vi "SMR_LabVIEW_V7.3.vi"() -> ()   [LabVIEW 2025]
uses:
  <vilib>/DAQmx/write.llb/DAQmx Write (Analog DBL 1Chan 1Samp).vi
  <vilib>/DAQmx/read.llb/DAQmx Read (Analog 1D DBL NChan 1Samp).vi
  <vilib>/DAQmx/create/channels.llb/DAQmx Create Channel (AI-Temperature-Thermocouple).vi
  <vilib>/DAQmx/create/channels.llb/DAQmx Create Channel (AI-Voltage-Basic).vi
  <vilib>/DAQmx/create/channels.llb/DAQmx Create Channel (AO-Voltage-Basic).vi
  <vilib>/DAQmx/miscellaneous.llb/DAQmx Fill In Error Info.vi
  <vilib>/addons/control/pid/pid.llb/PID (DBL).vi
  <vilib>/addons/control/pid/NI_PID_pid.lvlib
panel:
  out "Current Run Folder":path
  in  "Log Root Folder":path=path "C:/Users/LocalUser/Documents/GitHub/thermal-loop/resources/v0.1.1/data/001"
  out "Raw NI9201 \nVoltage Display":T1
  in  "Loop Period (ms)":dbl=1000.0
  in  "Stop":bool
  out "Auto Steady State Threshold (deg C/min)":dbl
  out "Max dT/dt (deg C/min)":dbl
  out "Temp Change Rate (deg C/min)":dbl
  out "5-Min Baseline Complete":bool
  out "Rate Window Ready":bool
  out "Steady State":bool
  in  "Voltage Limit (V)":dbl=10.0
  in  "Temperature Limit (C)":dbl=50.0
  in  "Pressure Limit (psi)":dbl=15.0
  out "Max Voltage":bool
  out "Max Temperature":bool
  out "Max Pressure":bool
  out "Heat Exchanger Pressure History":dbl(graph)
  out "Main Loop Pressure History":T2(graph)
  out "Overall Avg Pressure (psi)":dbl
  out "Heat Exchanger Pressure P6 (psi)":dbl
  out "Main Loop Avg Pressure (psi)":dbl
  out "Pressure Display":T3
  out "Overall Pressure History":T4(graph)
  out "Max Loop Pressure (psi)":dbl
  out "Heat Exchanger Temperature History":cluster{"Waveform":dbl, "Waveform":dbl}(graph)
  out "Main Loop Temeperature History":T5(graph)
  out "Heat Exchanger Avg Temp (deg C)":dbl
  out "Temperature Display":T6
  out "Overall Temperature History":T7(graph)
  out "Overall Avg Temp (deg C)":dbl
  out "Max Loop Temp (deg C)":dbl
  out "Final P-Valve Voltage (V)":dbl
  out "PID Trim Voltage (V)":dbl
  in  "PID Temp Setpoint (deg C)":dbl
  in  "Auto PID Enable":bool
  in  "Manual P-Valve Voltage (V)":dbl min=0.0 max=10.0
  out "Main Loop Avg Temp (deg C)":dbl
  in  "Flow Offset Correction (GPM)":dbl=-0.3
  out "Flow History":dbl(graph)
  out "Heat Exchanger Flow (GPM)":dbl
  # "Control/Troubleshoot"
  # "Steady State"
  # "Emergency Indicators"
  # "Pressure"
  # "Temperature"
  # "Proportional Valve Control"
  # "Heat Exchanger Flow"
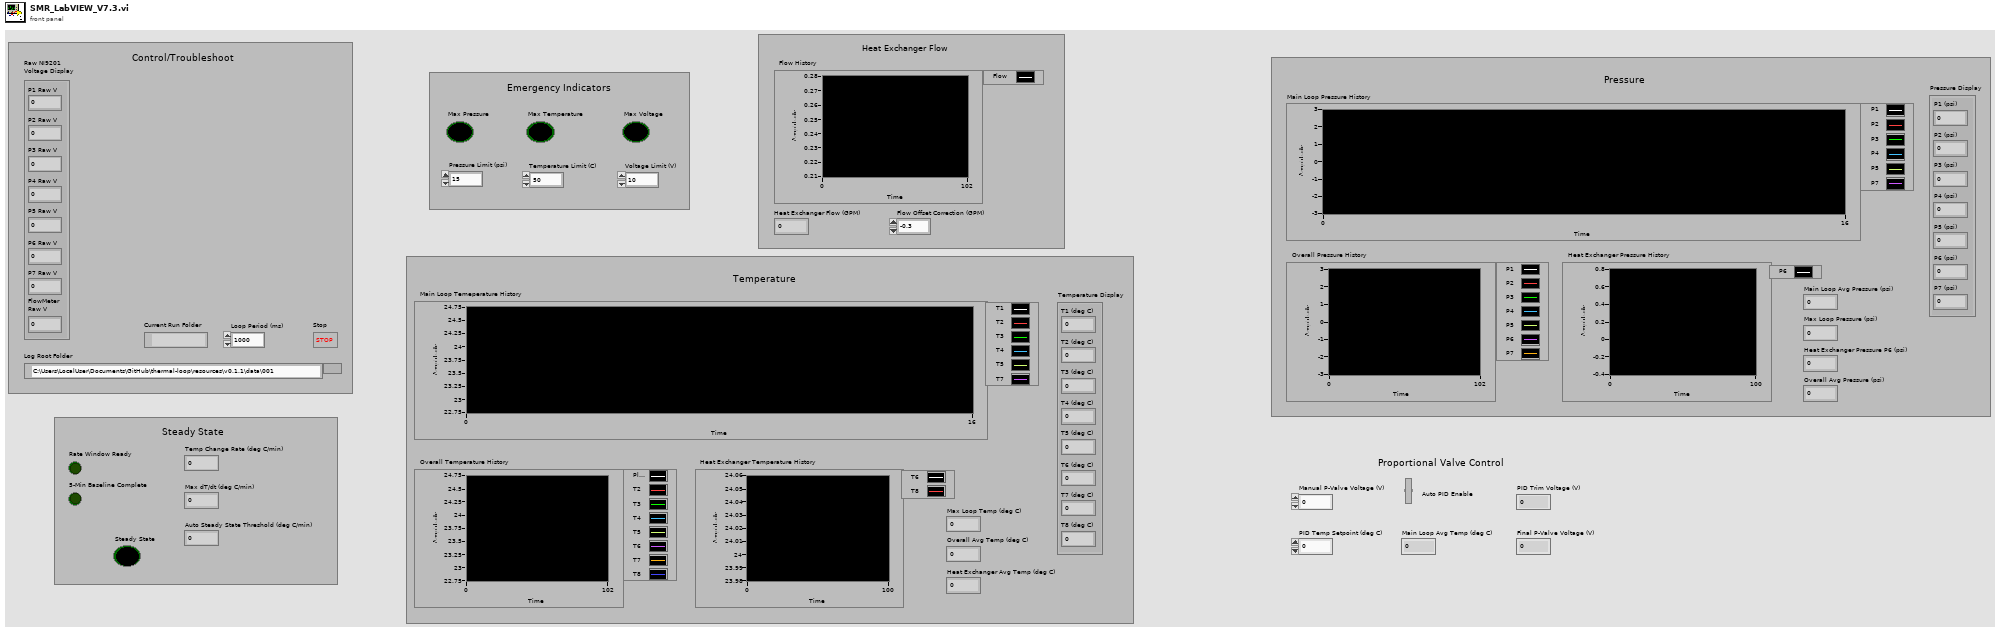
[diagram p1: front panel]
types:
  T1 = cluster{"P1 Raw V":dbl, "P2 Raw V":dbl, "P3 Raw V":dbl, "P4 Raw V":dbl, "P5 Raw V":dbl, "P6 Raw V":dbl, "P7 Raw V":dbl, "FlowMeter\nRaw V":dbl}
  T2 = cluster{"P1":dbl, "P2":dbl, "P3":dbl, "P4":dbl, "P5":dbl, "P7":dbl}
  T3 = cluster{"P1 (psi)":dbl, "P2 (psi)":dbl, "P3 (psi)":dbl, "P4 (psi)":dbl, "P5 (psi)":dbl, "P6 (psi)":dbl, "P7 (psi)":dbl}
  T4 = cluster{"P1":dbl, "P2":dbl, "P3":dbl, "P4":dbl, "P5":dbl, "P6":dbl, "P7":dbl}
  T5 = cluster{"Waveform":dbl, "Waveform":dbl, "Waveform":dbl, "Waveform":dbl, "Waveform":dbl, "Waveform":dbl}
  T6 = cluster{"T1 (deg C)":dbl, "T2 (deg C)":dbl, "T3 (deg C)":dbl, "T4 (deg C)":dbl, "T5 (deg C)":dbl, "T6 (deg C)":dbl, "T7 (deg C)":dbl, "T8 (deg C)":dbl}
  T7 = cluster{"Waveform":dbl, "Waveform":dbl, "Waveform":dbl, "Waveform":dbl, "Waveform":dbl, "Waveform":dbl, "Waveform":dbl, "Waveform":dbl}
  T8 = enum16{"open", "replace", "create", "open or create", "replace or create", "replace or create with confirmation"}
  T9 = cluster{"proportional gain (Kc)":dbl, "integral time (Ti, min)":dbl, "derivative time (Td, min)":dbl}
  T10 = cluster{"P1":dbl, "P2":dbl, "P3":dbl, "P4":dbl, "P5":dbl, "P6":dbl, "P7":dbl, "Flow":dbl}
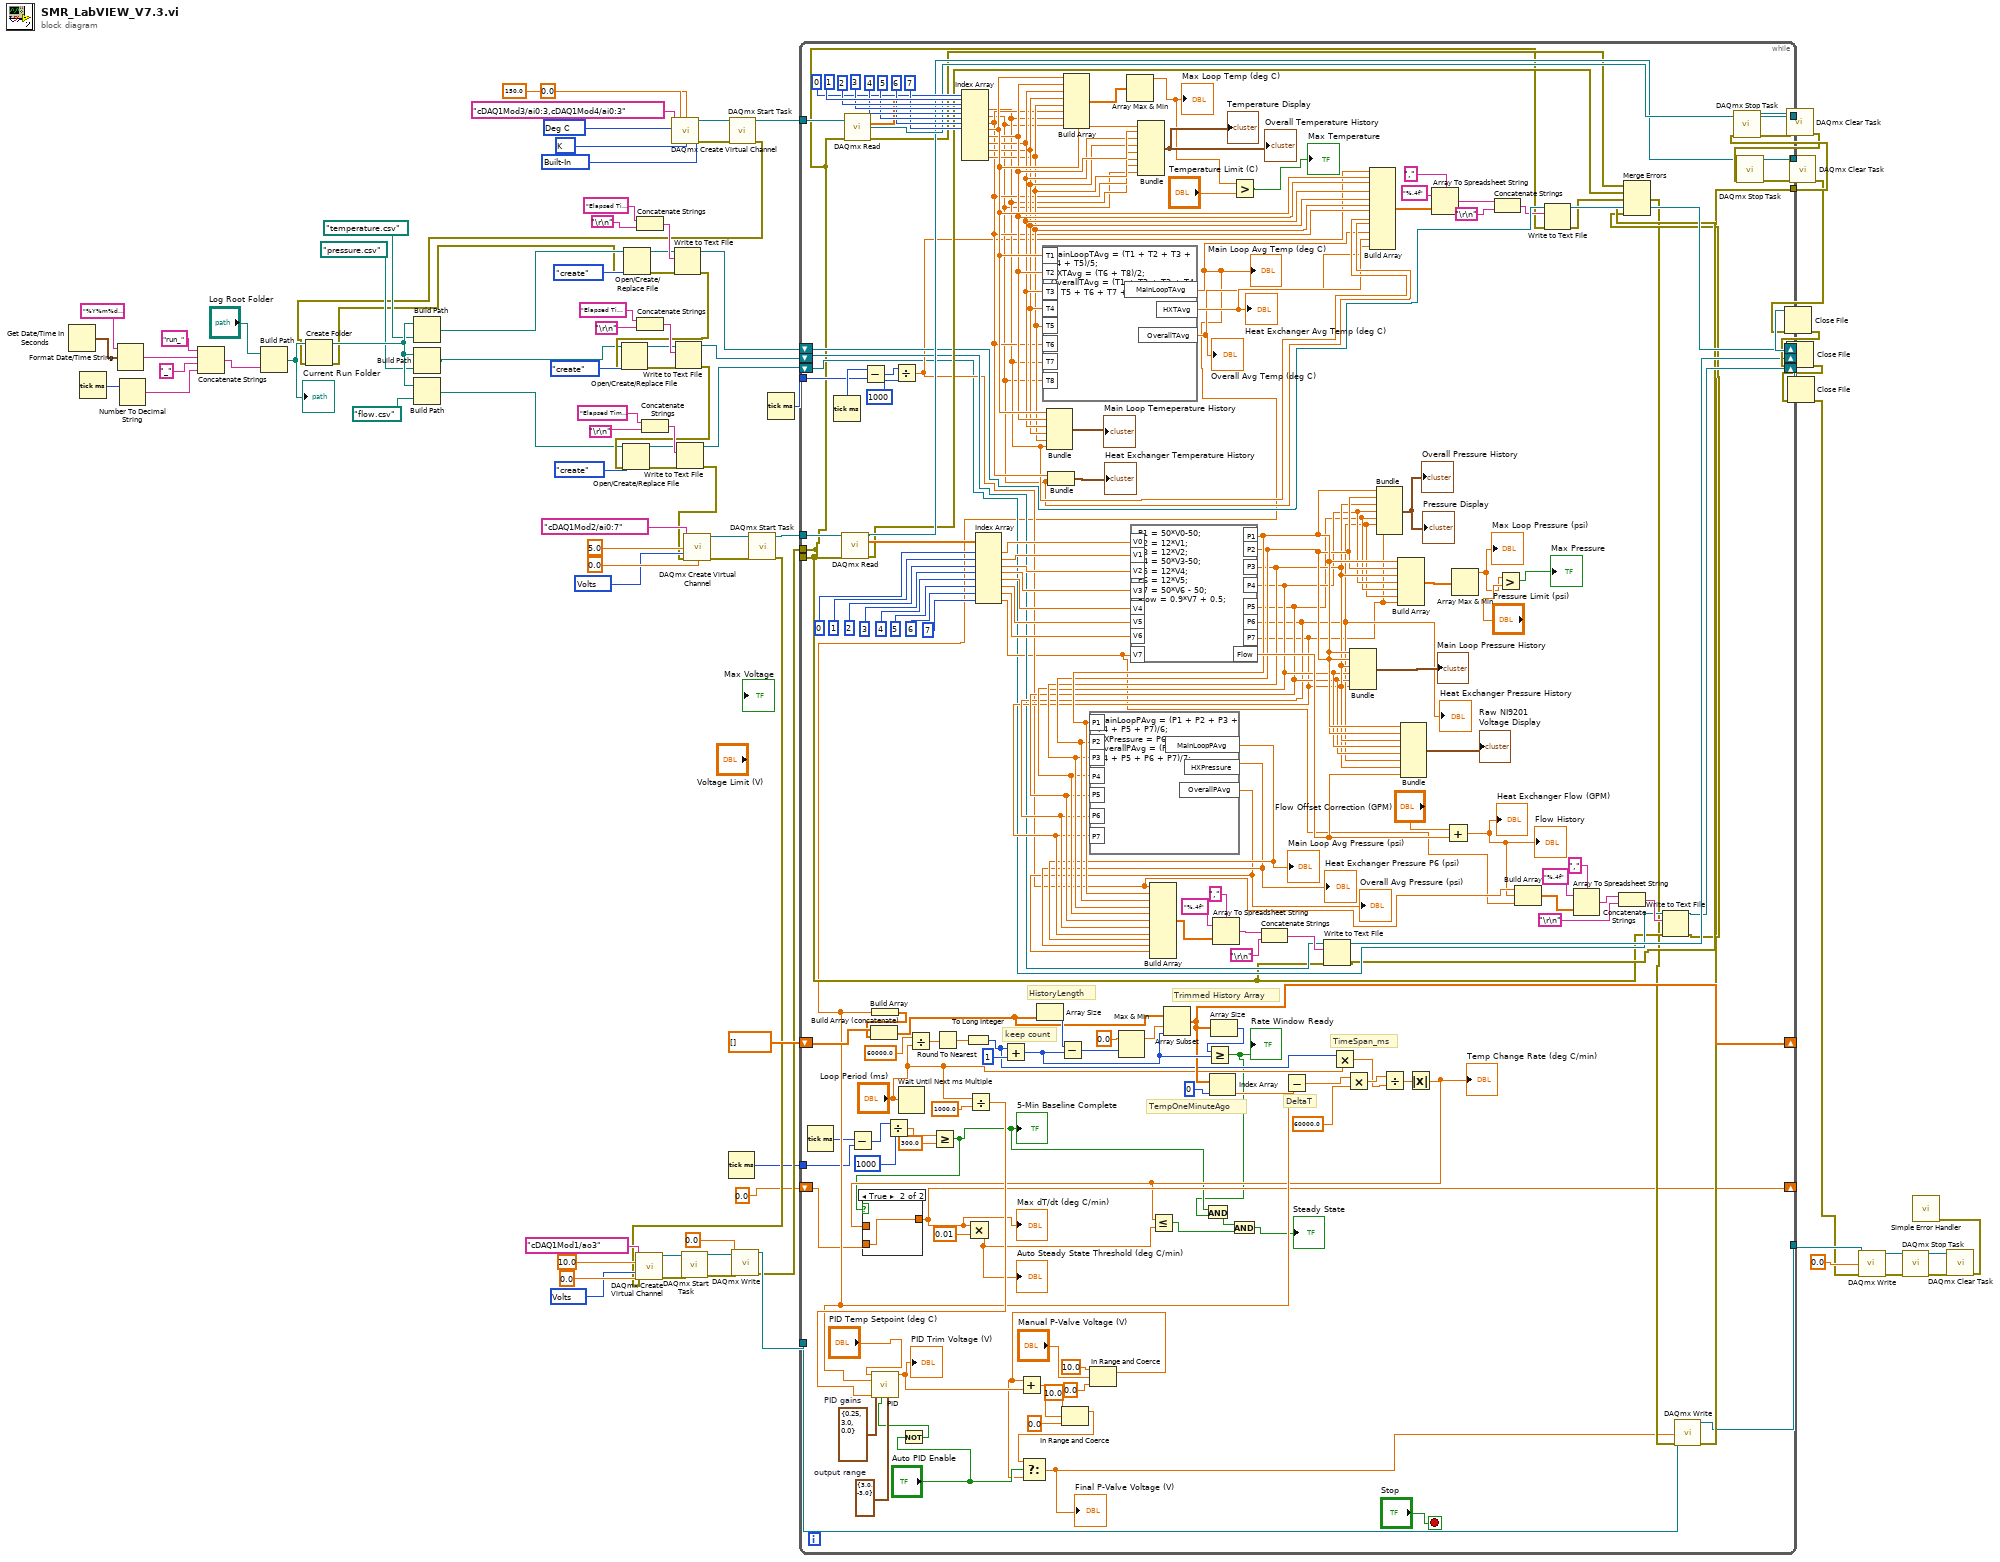
[diagram p0: block diagram]
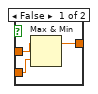
[diagram p2: hidden frame]
diagram:
  w19 = 10348 items=["Volts"=10348, "From Custom Scale"=10065] ("units")
  w85 = 10200 items=["Built-In"=10200, "Constant Value"=10116, "Channel"=10113] ("cjc source")
  w86 = 10073 items=["J"=10072, "K"=10073, "N"=10077, "R"=10082, "S"=10085, "T"=10086, "B"=10047, "E"=10055] ("thermocouple type")
  w87 = 10143 items=["Deg C"=10143, "Deg F"=10144, "Kelvins"=10325, "Deg R"=10145, "From Custom Scale"=10065] ("units")
  w94 = 10348 items=["Volts"=10348, "From Custom Scale"=10065] ("units")
  n1 = Get Date/Time In Seconds() -> (seconds since 1Jan1904=w42:timestamp)
  n2 = Tick Count (ms)() -> (millisecond timer value=w40:u32)
  n3 = Format Date/Time String(time format string (%c)="%Y%m%d_%H%M%S", seconds (now)=w42) -> (date/time string=w37:string)  [unwired: 1 in]
  n4 = Number To Decimal String(number=w40) -> (decimal integer string=w38:string)  [unwired: 1 in]
  n5 = Concatenate Strings("run_" ("string"), w37, "_" ("string"), w38) -> (w34:string)
  n6 = Build Path(base path="Log Root Folder", name or relative path=w34) -> (appended path=w33:path)
  "Current Run Folder" <- w33
  n7 = Concatenate Strings("Elapsed Time (s),T1 (deg C),T2 (deg C),T3 (deg C),T4 (deg C),T5 (deg C),T6 (deg C),T7 (deg C),T8 (deg C),Main Loop Avg Temp (deg C),HX Avg Temp (deg C),Overall Avg Temp (deg C)", "\r\n") -> (w68:string)
  n8 = Concatenate Strings("Elapsed Time (s),P1 (psi),P2 (psi),P3 (psi),P4 (psi),P5 (psi),P6 (psi),P7 (psi),Main Loop Avg Pressure (psi),HX Pressure (psi),Overall Avg Pressure (psi)", "\r\n") -> (w66:string)
  n9 = Concatenate Strings("Elapsed Time (s),Heat Exchanger Flow (GPM),Flow Raw Voltage (V)", "\r\n") -> (w62:string)
  n10 = call-poly <vilib>:"DAQmx Create Virtual Channel.vi"("maximum value"=150.0, "minimum value"=0.0, "physical channels"=tag "cDAQ1Mod3/ai0:3,cDAQ1Mod4/ai0:3", "cjc source"=w85, "units"=w87, "thermocouple type"=w86) -> ("task out"=w84:refnum<k21>, "error out"=w83:errorcluster)  [unwired: 8 in]
  n11 = Tick Count (ms)() -> (millisecond timer value=w2:u32)
  n12 = call <vilib>:"DAQmx Start Task.vi"("task/channels in"=w84, "error in"=w83) -> ("task out"=w82:refnum<k21>, "error out"=w25:errorcluster)  [unwired: 12 in]
  n13 = Create Folder(path (use dialog)=w33, error in=w25) -> (created path=w32:path, error out=w24:errorcluster)  [unwired: 1 in, 1 out]
  n14 = Build Path(base path=w32, name or relative path=path "temperature.csv") -> (appended path=w31:path)
  n15 = Build Path(base path=w32, name or relative path=path "pressure.csv") -> (appended path=w30:path)
  n16 = Build Path(base path=w32, name or relative path=path "flow.csv") -> (appended path=w29:path)
  n17 = Open/Create/Replace File(file path (use dialog)=w31, error in=w24, operation (0:open)=T8."create") -> (refnum out=w67:refnum<file>, error out=w51:errorcluster)  [unwired: 3 in, 1 out]
  n18 = Write to Text File(file (use dialog)=w67, text=w68, error in=w51) -> (refnum out=w58:refnum<file>, error out=w50:errorcluster)  [unwired: 1 in, 1 out]
  n19 = Open/Create/Replace File(file path (use dialog)=w30, error in=w50, operation (0:open)=T8."create") -> (refnum out=w65:refnum<file>, error out=w49:errorcluster)  [unwired: 3 in, 1 out]
  n20 = Write to Text File(file (use dialog)=w65, text=w66, error in=w49) -> (refnum out=w57:refnum<file>, error out=w48:errorcluster)  [unwired: 1 in, 1 out]
  n21 = Open/Create/Replace File(file path (use dialog)=w29, error in=w48, operation (0:open)=T8."create") -> (refnum out=w61:refnum<file>, error out=w47:errorcluster)  [unwired: 3 in, 1 out]
  n22 = Write to Text File(file (use dialog)=w61, text=w62, error in=w47) -> (refnum out=w56:refnum<file>, error out=w46:errorcluster)  [unwired: 1 in, 1 out]
  n23 = call-poly <vilib>:"DAQmx Create Virtual Channel.vi"("maximum value"=5.0, "minimum value"=0.0, "physical channels"=tag "cDAQ1Mod2/ai0:7", "units"=w94, "error in"=w46) -> ("task out"=w93:refnum<k21>, "error out"=w92:errorcluster)  [unwired: 9 in]
  n24 = call <vilib>:"DAQmx Start Task.vi"("task/channels in"=w93, "error in"=w92) -> ("task out"=w91:refnum<k21>, "error out"=w12:errorcluster)  [unwired: 12 in]
  n25 = call-poly <vilib>:"DAQmx Create Virtual Channel.vi"("maximum value"=10.0, "minimum value"=0.0, "physical channels"=tag "cDAQ1Mod1/ao3", "units"=w19, "error in"=w12) -> ("task out"=w18:refnum<k21>, "error out"=w17:errorcluster)  [unwired: 9 in]
  n26 = call <vilib>:"DAQmx Start Task.vi"("task/channels in"=w18, "error in"=w17) -> ("task out"=w16:refnum<k21>, "error out"=w15:errorcluster)  [unwired: 12 in]
  n27 = call-poly <vilib>:"DAQmx Write.vi"("task/channels in"=w16, "data"=0.0, "error in"=w15) -> ("task out"=w13:refnum<k21>, "error out"=w11:errorcluster)  [unwired: 10 in, 1 out]
  n28 = Tick Count (ms)() -> (millisecond timer value=w55:u32)
  n29 = while {
    tunnel: w91 -> [w259]
    tunnel: w82 -> [w233]
    tunnel: [w223] -> w81
    tunnel: [w134] -> _
    tunnel: [w222] -> w80
    tunnel: [w132] -> w79
    shift-right: [w199] -> w54
    shift-left: w58 -> [w200]
    shift-right: [w180] -> w53
    shift-left: w57 -> [w181]
    shift-right: [w169] -> w52
    shift-left: w56 -> [w170]
    tunnel: w55 -> [w218]
    shift-right: [w146] -> _
    shift-left: dbl[] [] -> [w159]
    tunnel: w13 -> [w124]
    tunnel: w11 -> [w134]
    tunnel: [w131] -> w9
    tunnel: w2 -> [w112]
    shift-right: [w105] -> _
    shift-left: 0.0 -> [w107]
    stop <- "Stop" stop-if-true
    w129 = cluster{"output high":dbl, "output low":dbl} {"output high"=3.0, "output low"=-3.0}  # output range
    w130 = T9 {"proportional gain (Kc)"=0.25, "integral time (Ti, min)"=3.0, "derivative time (Td, min)"=0.0}  # PID gains
    # "TimeSpan_ms"
    # "DeltaT"
    # "TempOneMinuteAgo"
    # "Trimmed History Array"
    # "HistoryLength"
    # "keep count"
    n30 = Tick Count (ms)() -> (millisecond timer value=w113:u32)
    n31 = Tick Count (ms)() -> (millisecond timer value=w219:u32)
    n32 = call-poly <vilib>:"DAQmx Read.vi"("task/channels in"=w259, "error in"=w134) -> ("task out"=w222:refnum<k21>, "data"=w250:dbl[], "error out"=w220:errorcluster)  [unwired: 11 in]
    n33 = call-poly <vilib>:"DAQmx Read.vi"("task/channels in"=w233, "error in"=w134) -> ("task out"=w223:refnum<k21>, "data"=w224:dbl[], "error out"=w221:errorcluster)  [unwired: 11 in]
    n34 = Subtract(x=w113, y=w112) -> (x-y=w111:u32)
    n35 = Subtract(x=w219, y=w218) -> (x-y=w217:u32)
    n36 = Divide(x=w111, y=u32 1000) -> (x/y=w109:dbl)
    n37 = Divide(x=w217, y=u32 1000) -> (x/y=w179:dbl)
    n38 = Wait Until Next ms Multiple(millisecond multiple="Loop Period (ms)") -> ()  [unwired: 1 out]
    n39 = Not(x="Auto PID Enable") -> (.not. x?=w125:bool)
    n40 = Divide(x=60000.0, y="Loop Period (ms)") -> (x/y=w156:dbl)
    n41 = Greater Or Equal?(x=w109, y=300.0) -> (x >= y?=w102:bool)
    "5-Min Baseline Complete" <- w102
    n42 = Round To Nearest(number=w156) -> (nearest integer value=w155:dbl)
    n43 = Index Array(array=w224, index #1=0 ("index"), index #2=1 ("index"), index #3=2 ("index"), index #4=3 ("index"), index #5=4 ("index"), index #6=5 ("index"), index #7=6 ("index"), index #8=7 ("index")) -> (element #1=w209:dbl, element #2=w208:dbl, element #3=w210:dbl, element #4=w215:dbl, element #5=w214:dbl, element #6=w213:dbl, element #7=w212:dbl, element #8=w211:dbl)
    n44 = To Long Integer(number=w155) -> (32bit integer=w143:i32)
    n45 = Divide(x="Loop Period (ms)", y=1000.0) -> (x/y=w126:dbl)
    n46 = Index Array(array=w250, index #1=0 ("index"), index #2=1 ("index"), index #3=2 ("index"), index #4=3 ("index"), index #5=4 ("index"), index #6=5 ("index"), index #7=6 ("index"), index #8=7 ("index")) -> (element #1=w249:dbl, element #2=w248:dbl, element #3=w247:dbl, element #4=w246:dbl, element #5=w245:dbl, element #6=w244:dbl, element #7=w243:dbl, element #8=w177:dbl)
    n47 = Add(x=w143, y=1) -> (x+y=w148:i32)
    n48 = formula code="MainLoopTAvg = (T1 + T2 + T3 + T4 + T5)/5;\nHXTAvg = (T6 + T8)/2;\nOverallTAvg = (T1 + T2 + T3 + T4 + T5 + T6 + T7 + T8)/8;"("T1"=w215, "T2"=w214, "T3"=w213, "T4"=w212, "T5"=w211, "T6"=w210, "T7"=w209, "T8"=w208) -> ("MainLoopTAvg"=w115:dbl, "HXTAvg"=w207:dbl, "OverallTAvg"=w206:dbl)
    "Overall Avg Temp (deg C)" <- w206
    "Main Loop Avg Temp (deg C)" <- w115
    "Heat Exchanger Avg Temp (deg C)" <- w207
    n49 = Build Array(w115) -> (w158:dbl[])
    n50 = Build Array (concatenate)(w159, w158) -> (w150:dbl[])
    n51 = call-poly <vilib>:"PID.vi"("reinitialize? (F)"=w125, "output range"=w129, "dt (s)"=w126, "PID gains"=w130, "process variable"=w115, "setpoint"="PID Temp Setpoint (deg C)") -> ("output"=w123:dbl)  [unwired: 4 in, 1 out]
    "PID Trim Voltage (V)" <- w123
    n52 = Array Size(array=w150) -> (size(s)=w153:i32)
    n53 = Bundle("Waveform"=w215, "Waveform"=w214, "Waveform"=w213, "Waveform"=w212, "Waveform"=w211, "Waveform"=w209) -> (→"Main Loop Temeperature History":T5)  [unwired: 1 in]
    n54 = Bundle("Waveform"=w210, "Waveform"=w208) -> (→"Heat Exchanger Temperature History":cluster{"Waveform":dbl, "Waveform":dbl})  [unwired: 1 in]
    n55 = Subtract(x=w153, y=w148) -> (x-y=w151:i32)
    n56 = Build Array(w215, w214, w213, w212, w211, w210, w209, w208) -> (w260:dbl[])
    n57 = In Range and Coerce(upper limit=10.0, x="Manual P-Valve Voltage (V)", lower limit=0.0) -> (coerced(x)=w118:dbl)  [unwired: 1 out]
    n58 = Add(x=w118, y=w123) -> (x+y=w122:dbl)
    n59 = In Range and Coerce(upper limit=10.0, x=w122, lower limit=0.0) -> (coerced(x)=w117:dbl)  [unwired: 1 out]
    n60 = Select(t=w117, s="Auto PID Enable", f=w118) -> (s? t:f=w116:dbl)
    "Final P-Valve Voltage (V)" <- w116
    n61 = Max & Min(x=0.0, y=w151) -> (max(x,y)=w149:dbl)  [unwired: 1 out]
    n62 = Array Max & Min(array=w260) -> (max value=w162:dbl)  [unwired: 3 out]
    "Max Loop Temp (deg C)" <- w162
    n63 = formula code="P1 = 50*V0-50;\nP2 = 12*V1;\nP3 = 12*V2;\nP4 = 50*V3-50;\nP5 = 12*V4;\nP6 = 12*V5; \nP7 = 50*V6 - 50;\nFlow = 0.9*V7 + 0.5;"("V0"=w249, "V1"=w248, "V2"=w247, "V3"=w246, "V4"=w245, "V5"=w244, "V6"=w243, "V7"=w177) -> ("P1"=w198:dbl, "P2"=w197:dbl, "P3"=w196:dbl, "P4"=w195:dbl, "P5"=w194:dbl, "P6"=w193:dbl, "P7"=w192:dbl, "Flow"=w238:dbl)
    "Heat Exchanger Pressure History" <- w193
    n64 = formula code="MainLoopPAvg = (P1 + P2 + P3 + P4 + P5 + P7)/6;\nHXPressure = P6;\nOverallPAvg = (P1 + P2 + P3 + P4 + P5 + P6 + P7)/7;"("P1"=w198, "P2"=w197, "P3"=w196, "P4"=w195, "P5"=w194, "P6"=w193, "P7"=w192) -> ("MainLoopPAvg"=w191:dbl, "HXPressure"=w190:dbl, "OverallPAvg"=w189:dbl)
    "Overall Avg Pressure (psi)" <- w189
    "Heat Exchanger Pressure P6 (psi)" <- w190
    "Main Loop Avg Pressure (psi)" <- w191
    n65 = Bundle("Waveform"=w215, "Waveform"=w214, "Waveform"=w213, "Waveform"=w212, "Waveform"=w211, "Waveform"=w210, "Waveform"=w209, "Waveform"=w208) -> (→"Overall Temperature History" →"Temperature Display":T7)  [unwired: 1 in]
    n66 = Build Array(w179, w198, w197, w196, w195, w194, w193, w192, w191, w190, w189) -> (w188:dbl[])
    n67 = Array Subset(array=w150, index=w149, length=w148) -> (w146:dbl[])
    n68 = Index Array(array=w146, index=0) -> (element=w144:dbl)
    n69 = Array Size(array=w146) -> (size(s)=w147:i32)
    n70 = Greater Or Equal?(x=w147, y=w148) -> (x >= y?=w101:bool)
    "Rate Window Ready" <- w101
    n71 = And(x=w102, y=w101) -> (x .and. y?=w100:bool)
    n72 = Array To Spreadsheet String(delimiter (Tab)=",", array=w188, 3:"%.4f" ("format string")) -> (spreadsheet string=w184:string)
    n73 = Greater?(x=w162, y="Temperature Limit (C)") -> (0:→"Max Temperature":bool)
    n74 = Concatenate Strings(w184, "\r\n") -> (w182:string)
    n75 = Subtract(x=w115, y=w144) -> (x-y=w142:dbl)
    n76 = Write to Text File(file (use dialog)=w181, text=w182, error in=w134) -> (refnum out=w180:refnum<file>, error out=w167:errorcluster)  [unwired: 1 in, 1 out]
    n77 = Multiply(x=w143, y="Loop Period (ms)") -> (x*y=w139:dbl)
    n78 = Multiply(x=w142, y=60000.0) -> (x*y=w140:dbl)
    n79 = Bundle("P1"=w198, "P2"=w197, "P3"=w196, "P4"=w195, "P5"=w194, "P7"=w192) -> (→"Main Loop Pressure History":T2)  [unwired: 1 in]
    n80 = Build Array(w179, w215, w214, w213, w212, w211, w210, w209, w208, w115, w207, w206) -> (w205:dbl[])
    n81 = Bundle("P1"=w198, "P2"=w197, "P3"=w196, "P4"=w195, "P5"=w194, "P6"=w193, "P7"=w192) -> (→"Overall Pressure History" →"Pressure Display":T4)  [unwired: 1 in]
    n82 = Divide(x=w140, y=w139) -> (x/y=w138:dbl)
    n83 = Build Array(w198, w197, w196, w195, w194, w193, w192) -> (w241:dbl[])
    n84 = Bundle("P1"=w198, "P2"=w197, "P3"=w196, "P4"=w195, "P5"=w194, "P6"=w193, "P7"=w192, "Flow"=w238) -> (→"Raw NI9201 \nVoltage Display":T10)  [unwired: 1 in]
    n85 = Absolute Value(x=w138) -> (abs(x)=w104:dbl)
    "Temp Change Rate (deg C/min)" <- w104
    n86 = case shown="True" w102 {
      tunnel: w107 -> [w264 w265]
      tunnel: w104 -> [w263 _]
      tunnel: [w262 w265] -> w105
      frame False {
        n87 = Max & Min(x=w263, y=w264) -> (max(x,y)=w262:dbl)  [unwired: 1 out]
      }
      frame True {
      }
    }
    "Max dT/dt (deg C/min)" <- w105
    n88 = Multiply(x=w105, y=0.01) -> (x*y=w103:dbl)
    "Auto Steady State Threshold (deg C/min)" <- w103
    n89 = Less Or Equal?(x=w104, y=w103) -> (x <= y?=w99:bool)
    n90 = And(x=w100, y=w99) -> (x .and. y?=→"Steady State":bool)
    n91 = Array To Spreadsheet String(delimiter (Tab)=",", array=w205, 3:"%.4f" ("format string")) -> (spreadsheet string=w202:string)
    n92 = Add(x="Flow Offset Correction (GPM)", y=w238) -> (x+y=w178:dbl)
    "Heat Exchanger Flow (GPM)" <- w178
    "Flow History" <- w178
    n93 = Array Max & Min(array=w241) -> (max value=w164:dbl)  [unwired: 3 out]
    "Max Loop Pressure (psi)" <- w164
    n94 = Concatenate Strings(w202, "\r\n") -> (w185:string)
    n95 = Greater?(x=w164, y="Pressure Limit (psi)") -> (0:→"Max Pressure":bool)
    n96 = Build Array(w179, w178, w177) -> (w176:dbl[])
    n97 = Write to Text File(file (use dialog)=w200, text=w185, error in=w134) -> (refnum out=w199:refnum<file>, error out=w168:errorcluster)  [unwired: 1 in, 1 out]
    n98 = Array To Spreadsheet String(delimiter (Tab)=",", array=w176, 3:"%.4f" ("format string")) -> (spreadsheet string=w172:string)
    n99 = Concatenate Strings(w172, "\r\n") -> (w171:string)
    n100 = Write to Text File(file (use dialog)=w170, text=w171, error in=w134) -> (refnum out=w169:refnum<file>, error out=w166:errorcluster)  [unwired: 1 in, 1 out]
    n101 = Merge Errors(w221, w220, w168, w167, w166) -> (w133:errorcluster)
    n102 = call-poly <vilib>:"DAQmx Write.vi"("task/channels in"=w124, "data"=w116, "error in"=w133) -> ("task out"=w131:refnum<k21>, "error out"=w132:errorcluster)  [unwired: 10 in, 1 out]
  }
  n103 = call <vilib>:"DAQmx Stop Task.vi"("task/channels in"=w81, "error in"=w79) -> ("task out"=w78:refnum<k21>, "error out"=w76:errorcluster)  [unwired: 12 in]
  n104 = call <vilib>:"DAQmx Clear Task.vi"("task in"=w78, "error in"=w76) -> ("error out"=w75:errorcluster)  [unwired: 13 in]
  n105 = call <vilib>:"DAQmx Stop Task.vi"("task/channels in"=w80, "error in"=w75) -> ("task out"=w77:refnum<k21>, "error out"=w74:errorcluster)  [unwired: 12 in]
  n106 = call <vilib>:"DAQmx Clear Task.vi"("task in"=w77, "error in"=w74) -> ("error out"=w45:errorcluster)  [unwired: 13 in]
  n107 = Close File(refnum=w54, error in=w45) -> (error out=w44:errorcluster)  [unwired: 1 out]
  n108 = Close File(refnum=w53, error in=w44) -> (error out=w43:errorcluster)  [unwired: 1 out]
  n109 = Close File(refnum=w52, error in=w43) -> (error out=w8:errorcluster)  [unwired: 1 out]
  n110 = call-poly <vilib>:"DAQmx Write.vi"("task/channels in"=w9, "data"=0.0, "error in"=w8) -> ("task out"=w7:refnum<k21>, "error out"=w5:errorcluster)  [unwired: 10 in, 1 out]
  n111 = call <vilib>:"DAQmx Stop Task.vi"("task/channels in"=w7, "error in"=w5) -> ("task out"=w6:refnum<k21>, "error out"=w4:errorcluster)  [unwired: 12 in]
  n112 = call <vilib>:"DAQmx Clear Task.vi"("task in"=w6, "error in"=w4) -> ("error out"=w3:errorcluster)  [unwired: 13 in]
  n113 = call <vilib>:"Simple Error Handler.vi"("error in (no error)"=w3) -> ()  [unwired: 4 in, 5 out]
